vi "Load Initial Peels and Strategies.vi"(8 "error in (no error)":errorcluster, 11 "Platano in":refnum<class "Platano.lvclass">) -> (0 "error out":errorcluster, 1 "Peels":set{refnum<class "BananaPeel.lvclass">}(c389), 2 "Ephemeral Strategies":map{string, refnum<class "BananaPeel.lvclass">}(c390), 3 "Platano out":refnum<class "Platano.lvclass">)   [LabVIEW 2021, in "Bananas.lvlib" / "Platano.lvclass"]
uses:
  Platano.lvclass
  BananaPeel/BananaPeel.lvclass
  Requirements/RequirementMap.lvclass
  C:/Repositories/LVOS/Bananas/lv-src/Bananas/BananaPeel/BananaPeel.lvclass
  BananaPeel.Example/GUID.lvclass
  BananaPeel.Project/Project.lvclass
  <vilib>/LabVIEW Open Source Project/Data Manipulation/TypeDescriptor/TypeDescriptor_GetName.vi
  <vilib>/LabVIEW Open Source Project/Data Manipulation/TypeDescriptor/TypeDescriptor_GetType.vi
  <vilib>/LabVIEW Open Source Project/Data Manipulation/TypeDescriptor/TypeDescriptor_GetPString.vi
  <vilib>/LabVIEW Open Source Project/Data Manipulation/Variant/OpenVariant.lvlib
  Bananas.lvlib
  TraceabilityMatrix/TraceabilityMatrix.lvclass
  C:/Repositories/LVOS/Bananas/lv-src/Bananas/Requirements/RequirementMap.lvclass
  C:/Repositories/LVOS/Bananas/lv-src/Bananas/TraceabilityMatrix/TraceabilityMatrix.lvclass
  C:/Repositories/LVOS/Bananas/lv-src/Bananas/BananaPeel.Example/GUID.lvclass
  C:/Repositories/LVOS/Bananas/lv-src/Bananas/BananaPeel.Project/Project.lvclass
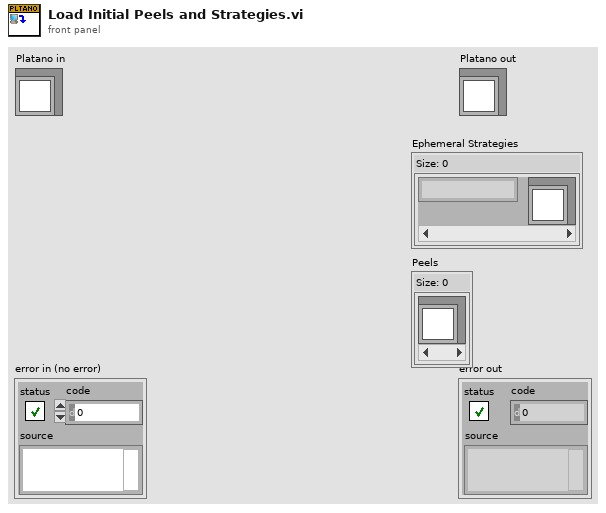
[diagram p1: front panel]
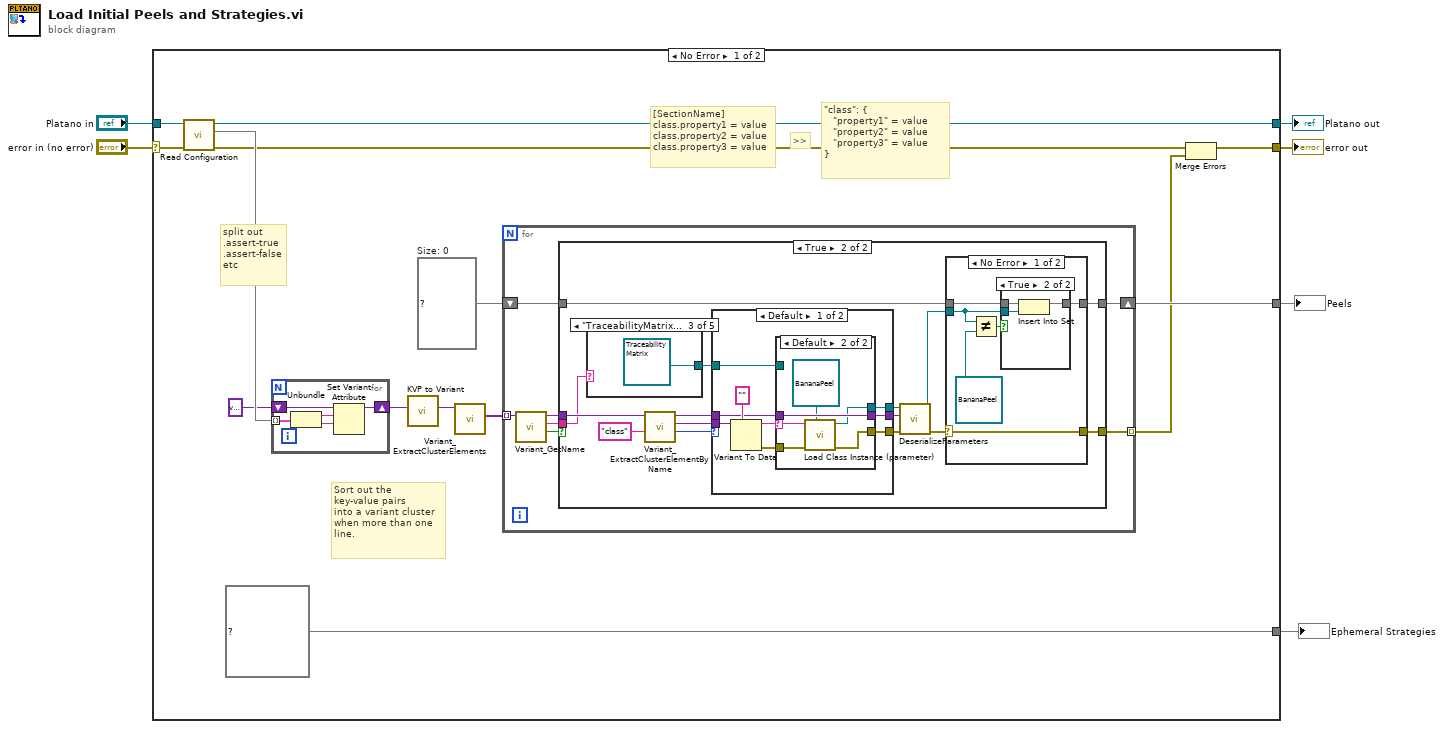
[diagram p0: block diagram]
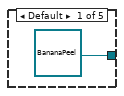
[diagram p7: hidden frame]
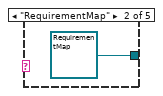
[diagram p8: hidden frame]
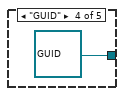
[diagram p9: hidden frame]
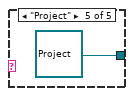
[diagram p10: hidden frame]
diagram:
  n1 = case shown="No Error" "error in (no error)" {
    selector: "error in (no error)" -> [w18 w86]
    tunnel: [w7 w86] -> w5
    tunnel: [w20 w85] -> w3
    tunnel: "Platano in" -> [w19 w85]
    tunnel: [w15 _] -> w2
    tunnel: [map{string, refnum<class "BananaPeel.lvclass">} {} ("Ephemeral Strategies") _] -> w1
    frame No Error {
      w17 = set{refnum<class "BananaPeel.lvclass">} {}  # Size: 0
      # "split out \n.assert-true\n.assert-false\netc"
      # ">>"
      # "\"class\": {\n   \"property1\" = value\n   \"property2\" = value\n   \"property3\" = value    \n}"
      # "[SectionName]\nclass.property1 = value\nclass.property2 = value\nclass.property3 = value"
      # "Sort out the\nkey-value pairs\ninto a variant cluster\nwhen more than one\nline."
      n2 = call "Read Configuration.vi"("error in (no error)"=w18, "Platano in"=w19) -> ("error out"=w8:errorcluster, "Config Map"=w14:map{string, string}, "Platano out"=w20:refnum<class "Platano.lvclass">)  [unwired: 7 in]
      n3 = for {
        tunnel: w14 -> [w25] mode=indexing
        shift-right: [w21] -> w12
        shift-left: variant -> [w24]
        n4 = Unbundle(w25) -> ("key"=w23:string, "value"=w22:string)
        n5 = Set Variant Attribute(Variant=w24, name=w23, value=w22) -> (Variant out=w21:variant)  [unwired: 1 in, 2 out]
      }
      n6 = call <vilib>:"KVP to Variant.vi"("KVP"=w12) -> ("Reconstructed Data"=w11:variant)  [unwired: 10 in]
      n7 = call <vilib>:"Variant_ExtractClusterElements.vi"("Cluster"=w11) -> ("Elements"=w10:variant[])  [unwired: 8 in, 2 out]
      n8 = for {
        shift-right: [w31] -> w15
        shift-left: w17 -> [w32]
        tunnel: w10 -> [w29] mode=indexing
        tunnel: [w28] -> w9 mode=indexing
        n9 = call <vilib>:"Variant_GetName.vi"("Variant"=w29) -> ("found"=w26:bool, "Name"=w27:string, "Variant dup"=w30:variant)  [unwired: 8 in]
        n10 = case shown="True" w26 {
          tunnel: w32 -> [w33 w48]
          tunnel: [w33 w47] -> w31
          tunnel: w30 -> [_ w46]
          tunnel: [_ w45] -> w28
          tunnel: w27 -> [_ w44]
          frame False {
          }
          frame True {
            n11 = case shown="\"TraceabilityMatrix\"" w44 {
              tunnel: [refnum<class "BananaPeel.lvclass"> refnum ("BananaPeel in") refnum<class "RequirementMap.lvclass"> refnum ("Bananas.lvlib:RequirementsMap.lvclass") refnum<class "TraceabilityMatrix.lvclass"> refnum ("Bananas.lvlib:TraceabilityMatrix.lvclass") refnum<class "GUID.lvclass"> refnum ("Bananas.lvlib:GUID.lvclass") refnum<class "Project.lvclass"> refnum ("Bananas.lvlib:Project.lvclass")] -> w43
              frame Default {
              }
              frame "RequirementMap" {
              }
              frame "TraceabilityMatrix" {
              }
              frame "GUID" {
              }
              frame "Project" {
              }
            }
            n12 = call <vilib>:"Variant_ExtractClusterElementByName.vi"("name"="class", "Cluster"=w46) -> ("index"=w41:i32, "Element"=w37:variant, "Cluster dup"=w38:variant)  [unwired: 7 in]
            n13 = case shown="Default" w41 {
              tunnel: [w66 w78] -> w40
              tunnel: [w62 w79] -> w39
              tunnel: w38 -> [w63 w79]
              tunnel: w37 -> [w69 _]
              tunnel: [w65 _] -> w34
              tunnel: w43 -> [w61 w78]
              frame Default {
                n14 = Variant To Data(type="", Variant=w69) -> (data=w64:string, error out=w67:errorcluster)  [unwired: 1 in]
                n15 = case shown="Default" w64 {
                  selector: w64 -> [_ w76]
                  tunnel: w67 -> [_ w75]
                  tunnel: [w70 w74] -> w66
                  tunnel: [_ w73] -> w65
                  tunnel: w63 -> [w71 w77]
                  tunnel: [w71 w77] -> w62
                  tunnel: w61 -> [w70 _]
                  frame "default" {
                  }
                  frame Default {
                    n16 = call "Load Class Instance (parameter).vi"("type"=refnum<class "BananaPeel.lvclass"> refnum ("BananaPeel in"), "error in"=w75, "parameter"=w76) -> ("error out"=w73:errorcluster, "specific class reference"=w74:refnum<class "BananaPeel.lvclass">)  [unwired: 7 in]
                  }
                }
              }
              frame -1 {
              }
            }
            n17 = call "DeserializeParameters.vi"("error in (no error)"=w34, "Variant"=w39, "BananaPeel in"=w40) -> ("error out"=w36:errorcluster, "BananaPeel out"=w35:refnum<class "BananaPeel.lvclass">)  [unwired: 7 in]
            n18 = case shown="No Error" w36 {
              selector: w36 -> [w52 w59]
              tunnel: w48 -> [w54 w60]
              tunnel: [w53 w60] -> w47
              tunnel: w35 -> [w50 _]
              tunnel: [w52 w59] -> w45
              frame No Error {
                n19 = Not Equal?(x=w50, y=refnum<class "BananaPeel.lvclass"> refnum ("BananaPeel in")) -> (x != y?=w49:bool)
                n20 = case shown="True" w49 {
                  tunnel: w54 -> [w55 w58]
                  tunnel: [w55 w57] -> w53
                  tunnel: w50 -> [_ w56]
                  frame False {
                  }
                  frame True {
                    n21 = Insert Into Set(10:w56, 11:w58) -> (3:w57:set{refnum<class "BananaPeel.lvclass">})  [unwired: 1 out]
                  }
                }
              }
              frame Error {
              }
            }
          }
        }
      }
      n22 = Merge Errors(w8, w9) -> (w7:errorcluster)
    }
    frame Error {
    }
  }
  "error out" <- w5
  "Platano out" <- w3
  "Ephemeral Strategies" <- w1
  "Peels" <- w2
